vi "RTK_Paths_Playground.vi"() -> ()   [LabVIEW 2014]
uses:
  <vilib>/Utility/file.llb/Read Delimited Spreadsheet (DBL).vi
panel:
  out "Array 2":string[][](array[string])
  out "Array":dbl[][](array[numeric])
  out "Relative Path from 1 to 2":path
  out "Common Path":path
  out "Path 2 Relative to Path 1?":bool
  out "All Files in Dir":path[](array[path])
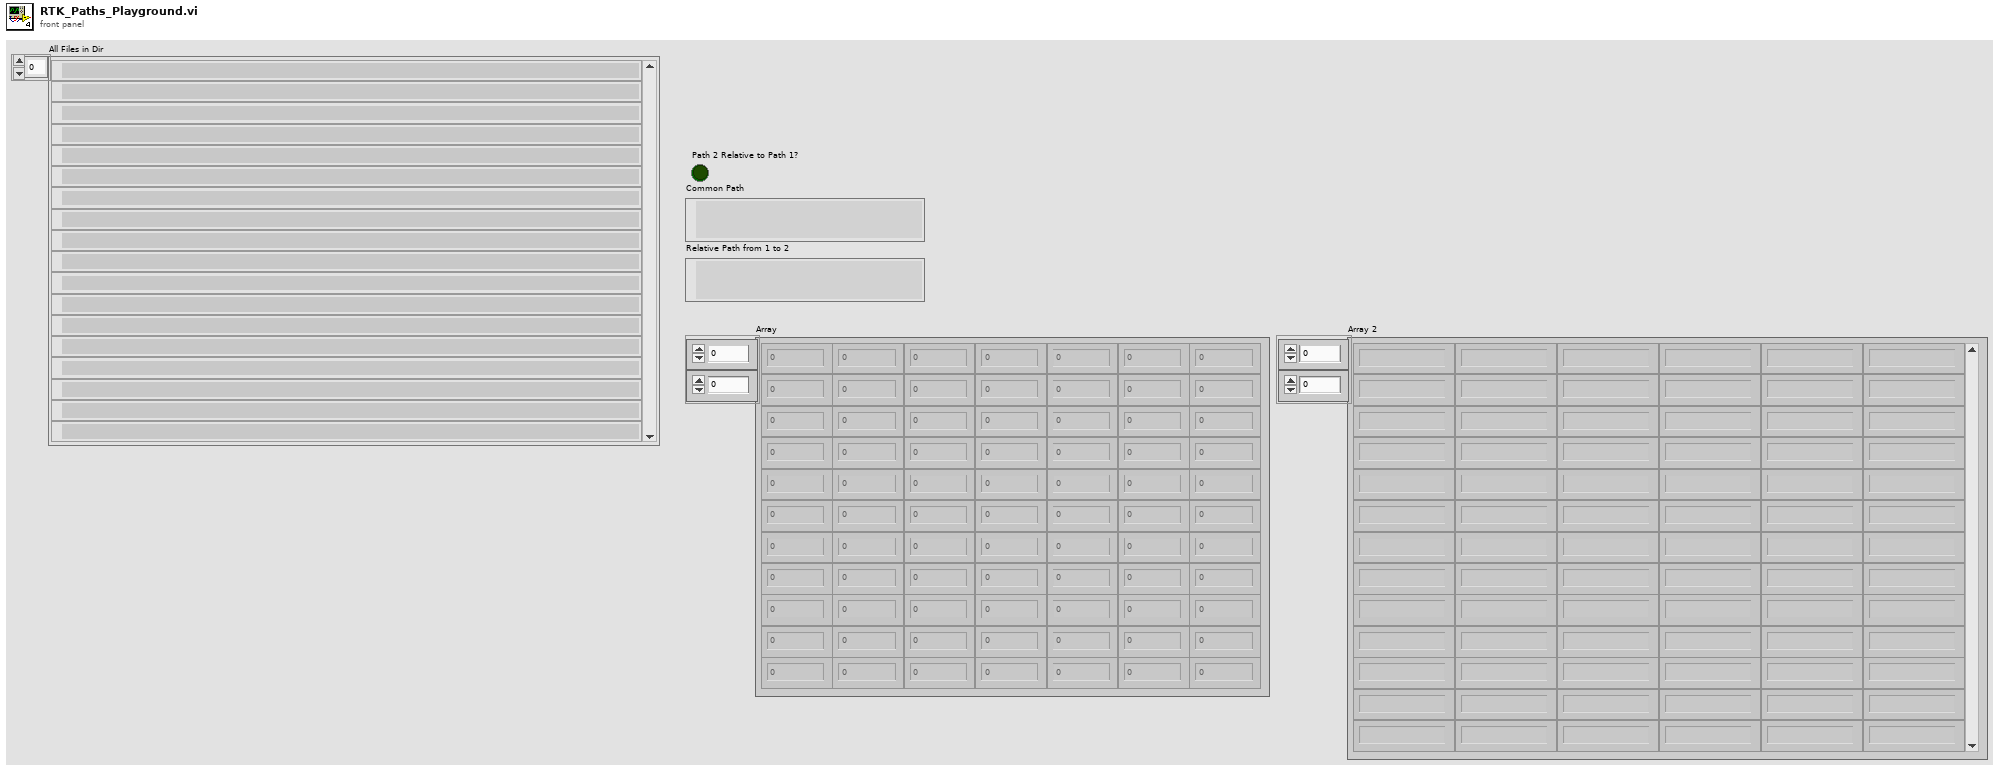
[diagram p1: front panel]
types:
  T1 = enum16{"whole column", "Value", "Max", "Min", "search Value", "etc"}[]
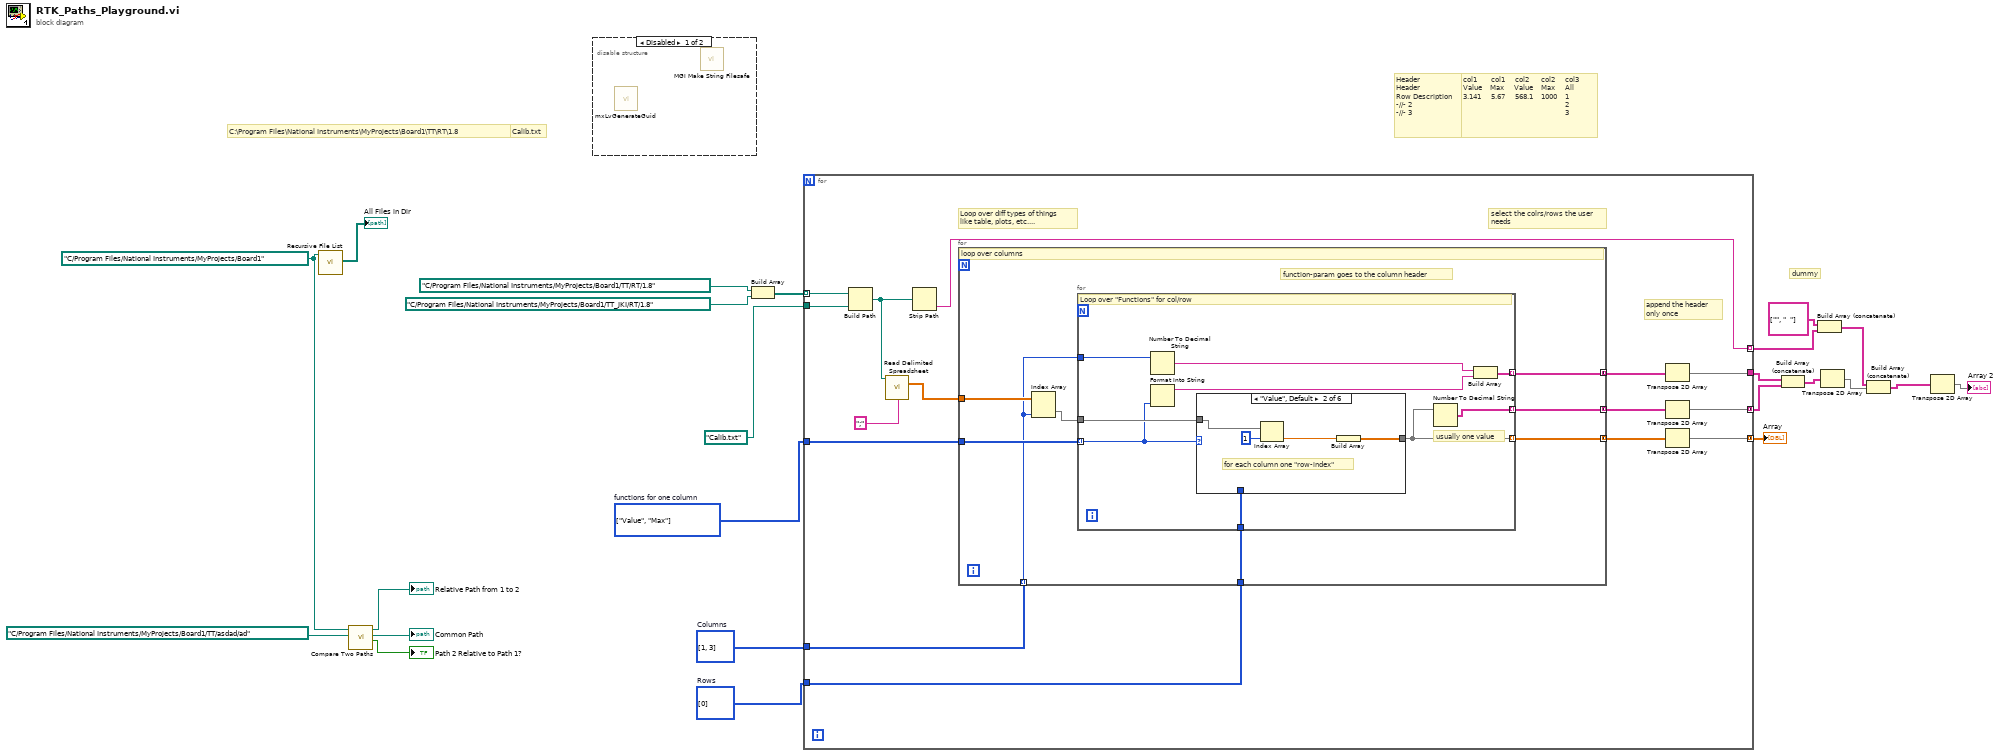
[diagram p0: block diagram]
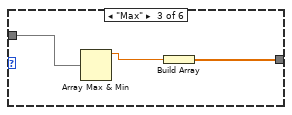
[diagram p3: hidden frame]
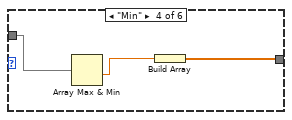
[diagram p4: hidden frame]
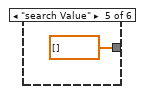
[diagram p5: hidden frame]
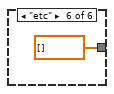
[diagram p6: hidden frame]
diagram:
  w10 = T1 [enum."Value", enum."Max"] items=["whole column", "Value", "Max", "Min", "search Value", "etc"]  # functions for one column
  w12 = i32[] [0]  # Rows
  w13 = i32[] [1, 3]  # Columns
  w22 = path "C:/Program Files/National Instruments/MyProjects/Board1" ("Folder Path")
  # "Header\nHeader\nRow Description\n-//- 2\n-//- 3"
  # "col1       col1     col2      col2     col3\nValue    Max     Value    Max     All\n3.141     5.67     568.1    1000    1\n                                                   2\n                                                   3"
  # "dummy"
  # "C:\\Program Files\\National Instruments\\MyProjects\\Board1\\TT\\RT\\1.8"
  # "Calib.txt"
  n1 = call <vilib>:"Recursive File List.vi"("Folder Path"=w22) -> ("All Files in Dir"=→"All Files in Dir":path[])  [unwired: 6 in, 4 out]
  n2 = call <vilib>:"Compare Two Paths.vi"("Path 2"=path "C:/Program Files/National Instruments/MyProjects/Board1/TT/asdad/ad" ("Folder Path"), "Path 1"=w22) -> ("Path 2 Relative to Path 1?"=→"Path 2 Relative to Path 1?":bool, "Common Path"=→"Common Path":path, "Relative Path from 1 to 2"=→"Relative Path from 1 to 2":path)  [unwired: 6 in, 1 out]
  n3 = disable-structure shown="Disabled" {
    frame Disabled {
      n4 = call <resource>:"mxLvGenerateGuid.vi"() -> ()  [unwired: 10 in, 2 out]
      n5 = call <userlib>:"MGI Make String Filesafe.vi"() -> ()  [unwired: 1 in, 1 out]
    }
    frame Enabled {
    }
  }
  n6 = Build Array(path "C:/Program Files/National Instruments/MyProjects/Board1/TT/RT/1.8" ("Folder Path"), path "C:/Program Files/National Instruments/MyProjects/Board1/TT_JKI/RT/1.8" ("Folder Path")) -> (w14:path[])
  n7 = for {
    tunnel: path "Calib.txt" ("Folder Path") -> [w38]
    tunnel: w14 -> [w37] mode=indexing
    tunnel: w13 -> [w35]
    tunnel: w12 -> [w34]
    tunnel: [w32] -> w11 mode=concatenating
    tunnel: w10 -> [w31]
    tunnel: [w27] -> w8 mode=concatenating
    tunnel: [w26] -> w9
    tunnel: [w24] -> w2 mode=indexing
    # "append the header\nonly once"
    # "select the colrs/rows the user\nneeds"
    # "Loop over diff types of things\nlike table, plots, etc...."
    n8 = Build Path(base path=w37, name or relative path=w38) -> (appended path=w25:path)
    n9 = call-poly <vilib>:"Read Delimited Spreadsheet.vi"("file path (dialog if empty)"=w25, "delimiter (\\t)"=";" ("delimiter (\\t)")) -> ("all rows"=w36:dbl[][])  [unwired: 8 in, 5 out]
    n10 = Strip Path(path=w25) -> (name=w24:string)  [unwired: 1 out]
    n11 = for {
      tunnel: w36 -> [w46]
      tunnel: w35 -> [w40] mode=indexing
      tunnel: w34 -> [w45]
      tunnel: [w42] -> w33 mode=concatenating
      tunnel: w31 -> [w43]
      tunnel: [w41] -> w29 mode=concatenating
      tunnel: [w39] -> w28 mode=concatenating
      # "function-param goes to the column header"
      # "loop over columns"
      n12 = Index Array(array=w46, index (col)=w40) -> (element=w44:dbl[])  [unwired: 1 in]
      n13 = for {
        tunnel: w45 -> [w55]
        tunnel: w44 -> [w54]
        tunnel: [w53] -> w42 mode=indexing
        tunnel: w43 -> [w52] mode=indexing
        tunnel: [w48] -> w41 mode=indexing
        tunnel: w40 -> [w50]
        tunnel: [w47] -> w39 mode=indexing
        # "usually one value"
        # "Loop over \"Functions\" for col/row"
        n14 = Number To Decimal String(number=w50) -> (decimal integer string=w49:string)  [unwired: 1 in]
        n15 = Format Into String(w52) -> (resulting string=w51:string)  [unwired: 3 in, 1 out]
        n16 = case shown="\"Value\", Default" w52 {
          tunnel: w55 -> [_ _ _ _ _ _]
          tunnel: w54 -> [w56 w60 w63 w66 _ _]
          tunnel: [w56 w57 w61 w65 dbl[] [] ("all rows") dbl[] [] ("all rows")] -> w53
          frame "whole column" {
          }
          frame "Value", Default {
            # "for each column one \"row-index\""
            n17 = Index Array(array=w60, index=1) -> (element=w58:dbl)
            n18 = Build Array(w58) -> (w57:dbl[])
          }
          frame "Max" {
            n19 = Array Max & Min(array=w63) -> (max value=w62:dbl)  [unwired: 3 out]
            n20 = Build Array(w62) -> (w61:dbl[])
          }
          frame "Min" {
            n21 = Array Max & Min(array=w66) -> (min value=w64:dbl)  [unwired: 3 out]
            n22 = Build Array(w64) -> (w65:dbl[])
          }
          frame "search Value" {
          }
          frame "etc" {
          }
        }
        n23 = Number To Decimal String(number=w53) -> (decimal integer string=w48:string[])  [unwired: 1 in]
        n24 = Build Array(w49, w51) -> (w47:string[])
      }
    }
    n25 = Transpose 2D Array(2D array=w28) -> (transposed array=w26:string[][])
    n26 = Transpose 2D Array(2D array=w29) -> (transposed array=w27:string[][])
    n27 = Transpose 2D Array(2D array=w33) -> (transposed array=w32:dbl[][])
  }
  "Array" <- w11
  n28 = Build Array (concatenate)(w9, w8) -> (w7:string[][])
  n29 = Build Array (concatenate)(string[] ["", "  "], w2) -> (w1:string[])
  n30 = Transpose 2D Array(2D array=w7) -> (transposed array=w6:string[][])
  n31 = Build Array (concatenate)(w1, w6) -> (w5:string[][])
  n32 = Transpose 2D Array(2D array=w5) -> (transposed array=→"Array 2":string[][])
